vi "FromUTMToObstacleSegments.vi"(1 "Input List of UTM locations to be arranged into segments":T1[](array[typedef]) {"North" format="%#_10f"; "East" format="%#_8f"}) -> (0 "Obstacle.lvclass":refnum<class "Obstacle.lvclass">)   [LabVIEW 2013, in "Obstacle.lvclass"]
doc: "Gets an input of a list of points, outputs an obstacle. Final segment is the last and first segments."
uses:
  Obstacle.lvclass
  Data/TypeDefs/UTM Location.ctl
  Obstacle.lvclass/Obstacle.ctl
panel:
  in  "Point Cluster":cluster{"Point 1":T1, "Point 0":T1} {"Point 0"."North" format="%#_10f"; "Point 0"."East" format="%#_8f"; "Point 1"."North" format="%#_10f"; "Point 1"."East" format="%#_8f"}
  in  "Obstacle.lvclass":refnum<class "Obstacle.lvclass">
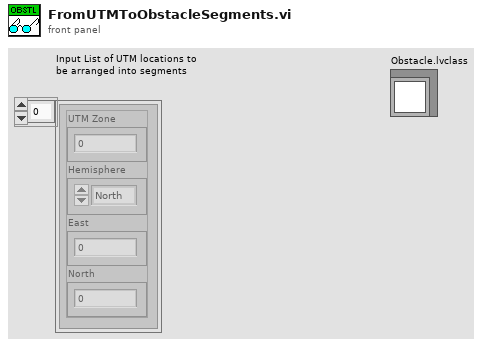
[diagram p1: front panel]
types:
  T1 = typedef "UTM Location.ctl" = cluster{"UTM Zone":dbl, "Hemisphere":enum16{"North", "South"}, "East":dbl, "North":dbl}
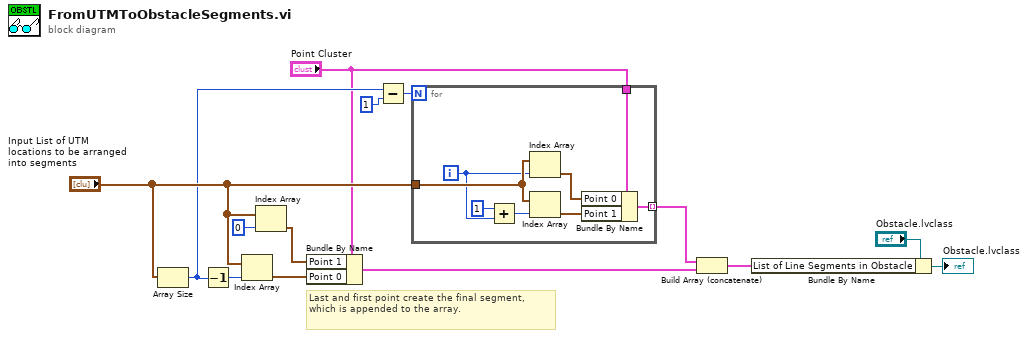
[diagram p0: block diagram]
diagram:
  # "Last and first point create the final segment, which is appended to the array."
  n1 = Array Size(array="Input List of UTM locations to be arranged into segments") -> (size(s)=w3:i32)
  n2 = Decrement(x=w3) -> (x-1=w2:i32)
  n3 = Index Array(array="Input List of UTM locations to be arranged into segments", index=w2) -> (element=w9:T1)
  n4 = Index Array(array="Input List of UTM locations to be arranged into segments", index=0) -> (element=w10:T1)
  n5 = Bundle By Name(cluster="Point Cluster", "Point 1"=w10, "Point 0"=w9) -> (w7:cluster{"Point 1":T1, "Point 0":T1})
  n6 = Subtract(x=w3, y=1) -> (x-y=w14:i32)
  n7 = for {
    N: w14 -> [_]
    tunnel: "Input List of UTM locations to be arranged into segments" -> [w22]
    tunnel: [w16] -> w8 mode=indexing
    tunnel: "Point Cluster" -> [w15]
    i -> [w19]
    n8 = Add(x=1, y=w19) -> (x+y=w21:i32)
    n9 = Index Array(array=w22, index=w19) -> (element=w18:T1)
    n10 = Index Array(array=w22, index=w21) -> (element=w17:T1)
    n11 = Bundle By Name(cluster=w15, "Point 0"=w18, "Point 1"=w17) -> (w16:cluster{"Point 1":T1, "Point 0":T1})
  }
  n12 = Build Array (concatenate)(w8, w7) -> (w6:cluster{"Point 1":T1, "Point 0":T1}[])
  n13 = Bundle By Name(cluster="Obstacle.lvclass", "List of Line Segments in Obstacle"=w6) -> (→"Obstacle.lvclass":refnum<class "Obstacle.lvclass">)
